vi "convertToKeyValuePair_example.vi"(8 "error in (no error)":errorcluster) -> (0 "error out":errorcluster)   [LabVIEW 2018]
doc: "Example of how to use Convert to Key Value Pair functions."
uses:
  convertToKeyValuePair_double.vi
  convertToKeyValuePair_integer.vi
  convertToKeyValuePair_boolean.vi
  convertToKeyValuePair_string.vi
  convertToKeyValuePair_1DArray.vi
  convertToKeyValuePair_2DArray.vi
panel:
  out "2D Array":string
  out "String":string
  out "1D Array":string
  out "Boolean":string
  out "Integer":string
  out "Double":string
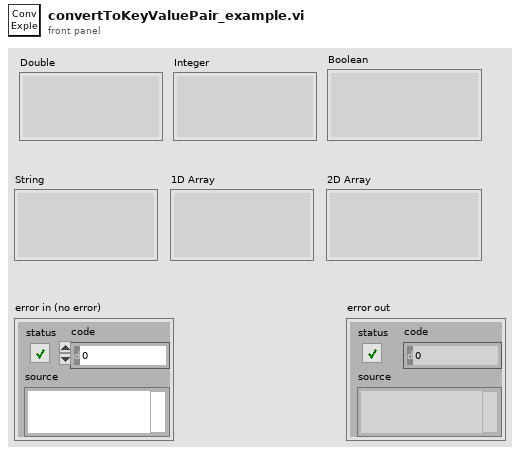
[diagram p1: front panel]
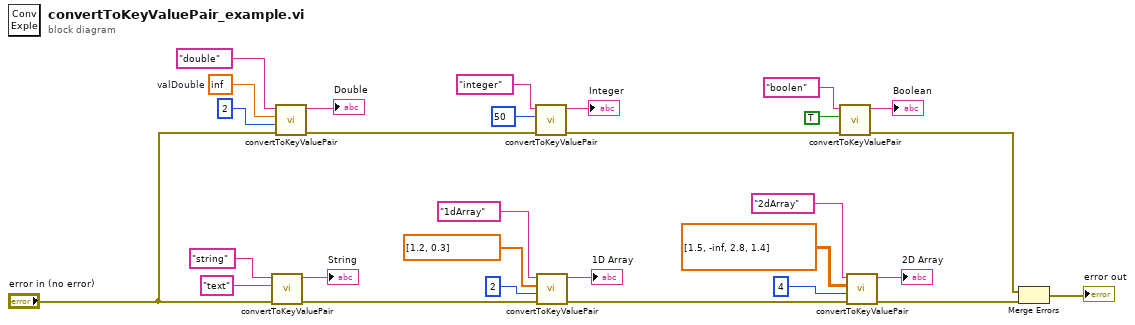
[diagram p0: block diagram]
diagram:
  w21 = inf  # valDouble
  n1 = call-poly "convertToKeyValuePair.vi"("error in (no error)"="error in (no error)", "value"="text", "name"="string") -> ("error out"=w8:errorcluster, "string converted"=→"String":string)  [unwired: 7 in]
  n2 = call-poly "convertToKeyValuePair.vi"("error in (no error)"="error in (no error)", "numZeros (0)"=u8 2 ("numZeros"), "value"=w21, "name"="double") -> ("error out"=w10:errorcluster, "string converted"=→"Double":string)  [unwired: 6 in]
  n3 = call-poly "convertToKeyValuePair.vi"("error in (no error)"=w10, "value"=50 ("valInteger"), "name"="integer") -> ("error out"=w9:errorcluster, "string converted"=→"Integer":string)  [unwired: 7 in]
  n4 = call-poly "convertToKeyValuePair.vi"("error in (no error)"=w8, "presicion (0)"=u8 2 ("numZeros"), "value"=dbl[] [1.2, 0.3], "name"="1dArray") -> ("error out"=w11:errorcluster, "string converted"=→"1D Array":string)  [unwired: 6 in]
  n5 = call-poly "convertToKeyValuePair.vi"("error in (no error)"=w9, "value"=TRUE, "name"="boolen") -> ("error out"=w5:errorcluster, "string converted"=→"Boolean":string)  [unwired: 7 in]
  n6 = call-poly "convertToKeyValuePair.vi"("error in (no error)"=w11, "presicion (0)"=u8 4 ("numZeros"), "value"=dbl[][] [[1.5, -inf], [2.8, 1.4]], "name"="2dArray") -> ("error out"=w6:errorcluster, "string converted"=→"2D Array":string)  [unwired: 6 in]
  n7 = Merge Errors(w5, w6) -> (→"error out":errorcluster)
